vi "APX VarianTMP L2.vi"() -> ()   [LabVIEW 2015]
uses:
  <vilib>/Instr/_visa.llb/VISA Configure Serial Port (Instr).vi
  <userlib>/caLab/Private/Get_PV-1D.vi
  <userlib>/caLab/Private/Put_DBL-1D_PV-1D.vi
  <userlib>/caLab/Private/Put_DBL_PV.vi
panel:
  out "AP2:L2TruboS":dbl
  out "TMPC5STRSTP 2":string
  out "APX:L2Turbo_STOP":bool
  out "APX:L2Turbo_START":bool
  out "TMPC5STRSTP":string
  out "SERIAL":string
  out "V-301":refnum<visa-resource-name>="COM4"
  out "APX:L2TurboF":dbl caption="F_20/Hz"
  out "APX:L2TurboP":dbl caption="P_20/W"
  out "APX:L2TurboS:STR":string
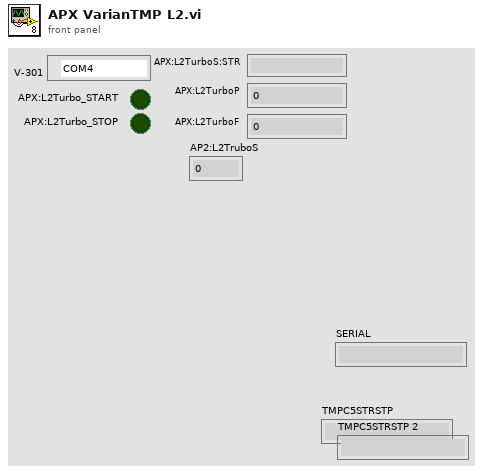
[diagram p1: front panel]
types:
  T1 = enum16{"START", "STOP", "REMOTE/SERIAL", "REMOTE", "SERIAL", "START/STOP", "PUMP STATUS", "Driving Frequency", "PUMP POWER", "PRESSURE"}
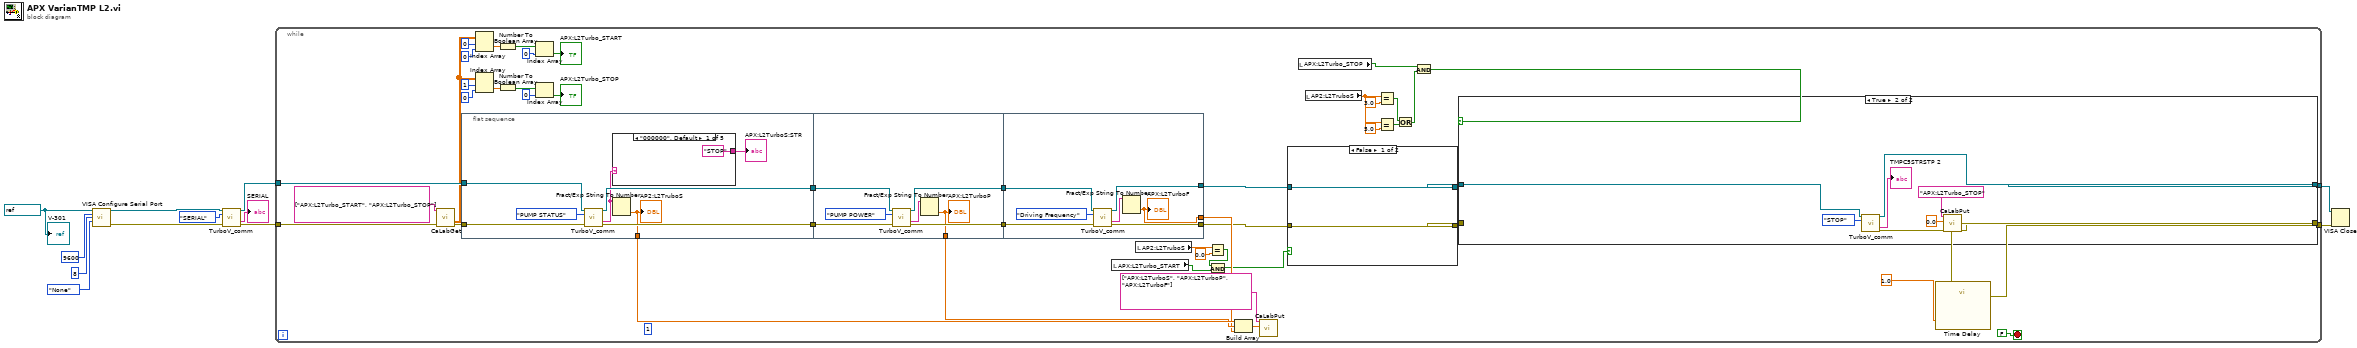
[diagram p0: block diagram]
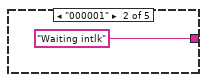
[diagram p2: hidden frame]
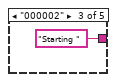
[diagram p3: hidden frame]
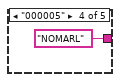
[diagram p4: hidden frame]
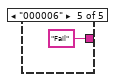
[diagram p5: hidden frame]
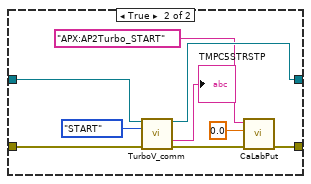
[diagram p7: hidden frame]
diagram:
  w12 = refnum<visa-resource-name> "COM4" ("VISA resource name")
  n1 = call-poly "VISA Configure Serial Port"("VISA resource name"=w12, "baud rate (9600)"=u32 9600, "data bits (8)"=u16 8, "parity (0:none)"=enum16{"None", "Odd", "Even", "Mark", "Space"}."None") -> ("VISA resource name out"=w5:refnum<visa-resource-name>, "error out"=w3:errorcluster)  [unwired: 10 in]
  n2 = call "TurboV_comm.vi"("VISA resource name"=w5, "Command"=T1."SERIAL", "error in (no error)"=w3) -> ("VISA resource name out"=w4:refnum<visa-resource-name>, "read buffer"=→"SERIAL":string, "error out"=w2:errorcluster)  [unwired: 10 in]
  n3 = while {
    tunnel: w4 -> [w60]
    tunnel: w2 -> [w39]
    tunnel: [w20] -> w8
    tunnel: [w58] -> w7
    stop <- FALSE stop-if-true
    (unwired) 1
    n4 = call-poly "CaLabGet.vi"("PV Names"=string[] ["APX:L2Turbo_START", "APX:L2Turbo_STOP"], "Error in (no error)"=w39) -> ("Value Array (number)"=w41:dbl[][], "Error out"=w40:errorcluster)  [unwired: 7 in, 5 out]
    n5 = flat-sequence {
      tunnel: w60 -> [w68]
      tunnel: w40 -> [w67]
      tunnel: [w66] -> w29
      tunnel: [w65] -> w28
      tunnel: [w61] -> w56
      tunnel: w29 -> [w79]
      tunnel: w28 -> [w76]
      tunnel: [w78] -> w27
      tunnel: [w77] -> w26
      tunnel: [w74] -> w55
      tunnel: w27 -> [w87]
      tunnel: w26 -> [w86]
      tunnel: [w83] -> w23
      tunnel: [w82] -> w24
      tunnel: [w81] -> w54
      frame #0 {
        n6 = call "TurboV_comm.vi"("VISA resource name"=w68, "Command"=T1."PUMP STATUS", "error in (no error)"=w67) -> ("VISA resource name out"=w66:refnum<visa-resource-name>, "read buffer"=w62:string, "error out"=w65:errorcluster)  [unwired: 10 in]
        n7 = case shown="\"000000\", Default" w62 {
          tunnel: ["STOP" "Waiting intlk" "Starting " "NOMARL" "Fail"] -> w63
          frame "000000", Default {
          }
          frame "000001" {
          }
          frame "000002" {
          }
          frame "000005" {
          }
          frame "000006" {
          }
        }
        "APX:L2TurboS:STR" <- w63
        n8 = Fract/Exp String To Number(string=w62) -> (number=w61:dbl)  [unwired: 3 in, 1 out]
        "AP2:L2TruboS" <- w61
      }
      frame #1 {
        n9 = call "TurboV_comm.vi"("VISA resource name"=w79, "Command"=T1."PUMP POWER", "error in (no error)"=w76) -> ("VISA resource name out"=w78:refnum<visa-resource-name>, "read buffer"=w75:string, "error out"=w77:errorcluster)  [unwired: 10 in]
        n10 = Fract/Exp String To Number(string=w75) -> (number=w74:dbl)  [unwired: 3 in, 1 out]
        "APX:L2TurboP" <- w74
      }
      frame #2 {
        n11 = call "TurboV_comm.vi"("VISA resource name"=w87, "Command"=T1."Driving Frequency", "error in (no error)"=w86) -> ("VISA resource name out"=w82:refnum<visa-resource-name>, "read buffer"=w84:string, "error out"=w83:errorcluster)  [unwired: 10 in]
        n12 = Fract/Exp String To Number(string=w84) -> (number=w81:dbl)  [unwired: 3 in, 1 out]
        "APX:L2TurboF" <- w81
      }
    }
    n13 = Index Array(array=w41, index (row)=0 ("disabled index (row)"), index (col)=0 ("index (row)")) -> (element=w47:dbl)
    n14 = Index Array(array=w41, index (row)=1 ("disabled index (row)"), index (col)=0 ("index (row)")) -> (element=w42:dbl)
    n15 = Number To Boolean Array(number=w47) -> (Boolean array=w49:bool[])
    n16 = Number To Boolean Array(number=w42) -> (Boolean array=w44:bool[])
    n17 = Index Array(array=w49, index=0) -> (element=→"APX:L2Turbo_START":bool)
    n18 = Index Array(array=w44, index=0) -> (element=→"APX:L2Turbo_STOP":bool)
    n19 = local read "APX:L2Turbo_START"() -> (w14:bool)
    n20 = local read "AP2:L2TruboS"() -> (w35:dbl)
    n21 = Equal?(x=w35, y=0.0) -> (x = y?=w16:bool)
    n22 = And(x=w16, y=w14) -> (x .and. y?=w15:bool)
    n23 = Build Array(w56, w55, w54) -> (w53:dbl[])
    n24 = call-poly <userlib>:"CaLabPut.vi"("Values"=w53, "PV Names"=string[] ["APX:L2TurboS", "APX:L2TurboP", "APX:L2TurboF"]) -> ()  [unwired: 6 in, 4 out]
    n25 = case shown="False" w15 {
      tunnel: [w99 w106] -> w22
      tunnel: [w98 w100] -> w21
      tunnel: w24 -> [w99 w105]
      tunnel: w23 -> [w98 w104]
      frame False {
      }
      frame True {
        n26 = call "TurboV_comm.vi"("VISA resource name"=w105, "Command"=T1."START", "error in (no error)"=w104) -> ("VISA resource name out"=w106:refnum<visa-resource-name>, "read buffer"=→"TMPC5STRSTP":string, "error out"=w101:errorcluster)  [unwired: 10 in]
        n27 = call-poly <userlib>:"CaLabPut.vi"("Error in (no error)"=w101, "Value"=0.0, "PV Name"="APX:AP2Turbo_START") -> ("Error out"=w100:errorcluster)  [unwired: 5 in, 3 out]
      }
    }
    n28 = local read "APX:L2Turbo_STOP"() -> (w19:bool)
    n29 = local read "AP2:L2TruboS"() -> (w34:dbl)
    n30 = Equal?(x=w34, y=3.0) -> (x = y?=w32:bool)
    n31 = Equal?(x=w34, y=5.0) -> (x = y?=w33:bool)
    n32 = Or(x=w32, y=w33) -> (x .or. y?=w18:bool)
    n33 = And(x=w19, y=w18) -> (x .and. y?=w17:bool)
    n34 = case shown="True" w17 {
      tunnel: [w89 w96] -> w20
      tunnel: [w88 w90] -> w13
      tunnel: w22 -> [w89 w95]
      tunnel: w21 -> [w88 _]
      frame False {
      }
      frame True {
        n35 = call "TurboV_comm.vi"("VISA resource name"=w95, "Command"=T1."STOP") -> ("VISA resource name out"=w96:refnum<visa-resource-name>, "read buffer"=→"TMPC5STRSTP 2":string, "error out"=w91:errorcluster)  [unwired: 11 in]
        n36 = call-poly <userlib>:"CaLabPut.vi"("Error in (no error)"=w91, "Value"=0.0, "PV Name"="APX:L2Turbo_STOP") -> ("Error out"=w90:errorcluster)  [unwired: 5 in, 3 out]
      }
    }
    n37 = call "Time Delay"("error in (no error)"=w13, "Delay Time (s)"=1.0) -> ("error out"=w58:errorcluster)  [unwired: 9 in]
  }
  n38 = VISA Close(VISA resource name=w8, error in (no error)=w7) -> ()  [unwired: 1 out]
  "V-301" <- w12
